vi "Read Steps From File.vi"(0 "Sequence Context":T2) -> (1 "Test Data":T1 {"Numeric Measurement" format="%.2f"}, 2 "error out":errorcluster)   [LabVIEW 2013]
uses:
  <vilib>/addons/TestStand/_TSLegacy.llb/LabVIEW Test - Sequence Context.ctl
  Demo/LabVIEW/SupportVIs.llb/LabVIEW Test - Test Data.ctl
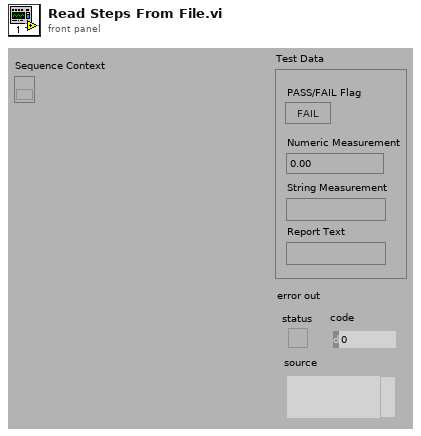
[diagram p1: front panel]
types:
  T1 = typedef "LabVIEW Test - Test Data.ctl" = cluster{"PASS/FAIL Flag":bool, "Numeric Measurement":dbl, "String Measurement":string, "Report Text":string}
  T2 = typedef "LabVIEW Test - Sequence Context.ctl" = refnum<k7>
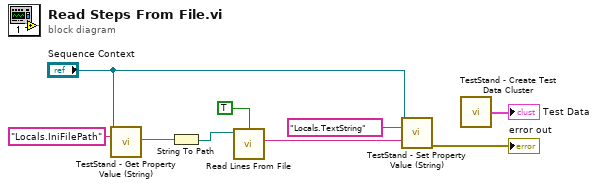
[diagram p0: block diagram]
diagram:
  n1 = call <vilib>:"TestStand - Get Property Value (String).vi"("Sequence Context In"="Sequence Context", "Lookup String"="Locals.IniFilePath") -> ("Value"=w3:string)  [unwired: 1 in, 12 out]
  n2 = String To Path(string=w3) -> (path=w4:path)
  n3 = call <vilib>:"Read Lines From File.vi"("convert eol? (no:F)"=TRUE, "file path (dialog if empty)"=w4) -> ("line string"=w6:string)  [unwired: 1 in, 6 out]
  n4 = call <vilib>:"TestStand - Set Property Value (String).vi"("Sequence Context In"="Sequence Context", "Lookup String"="Locals.TextString", "New Value"=w6) -> ("error out"=→"error out":errorcluster)  [unwired: 2 in, 10 out]
  n5 = call "TestStand - Create Test Data Cluster.vi"() -> ("Test Data"=→"Test Data":T1)  [unwired: 4 in]
